vi "load.vi"(8 "error in (no error)":errorcluster, 10 "Node":refnum<k20>, 11 "HP83623A_RF_Generator in":refnum<class "HP83623A_RF_Generator.lvclass">) -> (0 "error out":errorcluster, 2 "node out":refnum<k20>, 3 "HP83623A_RF_Generator out":refnum<class "HP83623A_RF_Generator.lvclass">)   [LabVIEW 2013, in "HP83623A_RF_Generator.lvclass"]
uses:
  HP83623A_RF_Generator.lvclass
  HP83623A.ctl
  HP83623A_RF_Generator.lvclass/HP83623A_RF_Generator.ctl
  <vilib>/xml/Close Reference(Node).vi
  <vilib>/xml/NI_XML.lvlib
  <resource>/objmgr/DOMUserDefRef.rc
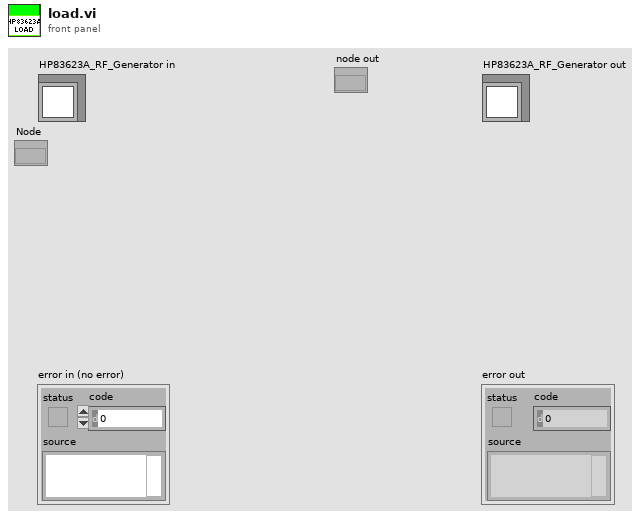
[diagram p1: front panel]
types:
  T1 = typedef "HP83623A_RF_Generator.lvclass/HP83623A.ctl" = cluster{"Frequency (Hz)":dbl, "Power (dBm)":dbl, "Enabled":bool, "initialized":bool, "RF Output On/Off":bool, "External Trigger?":bool, "VISA Session":refnum<visa-resource-name>, "Generator Name":string}
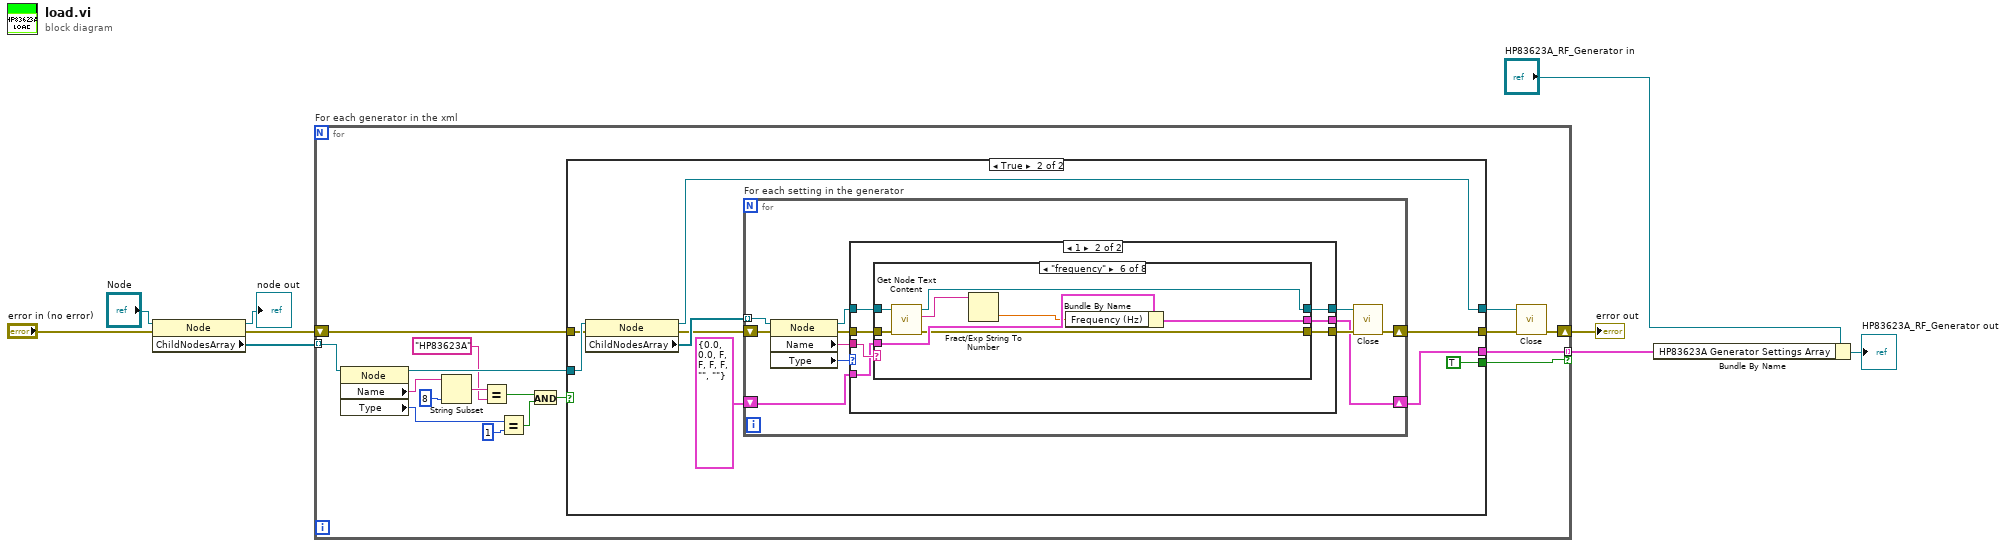
[diagram p0: block diagram]
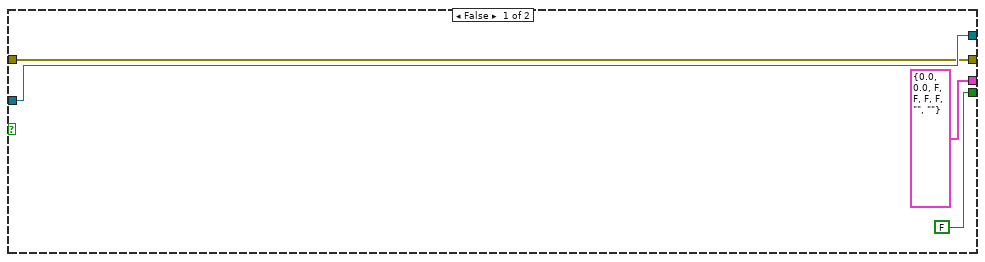
[diagram p2: hidden frame]
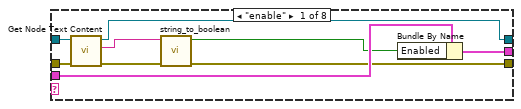
[diagram p4: hidden frame]
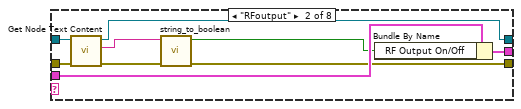
[diagram p5: hidden frame]
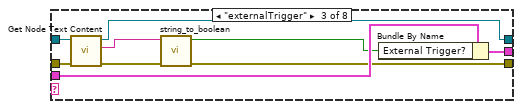
[diagram p6: hidden frame]
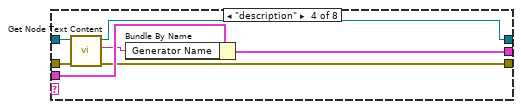
[diagram p7: hidden frame]
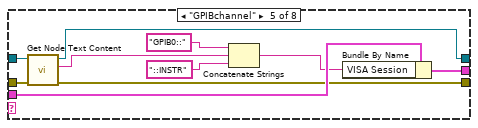
[diagram p8: hidden frame]
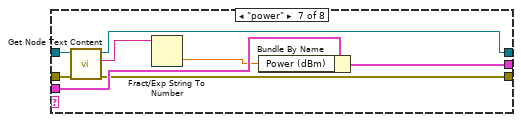
[diagram p9: hidden frame]
diagram:
  n1 = property class="Node"(reference="Node", error in="error in (no error)") -> (reference out=→"node out":refnum<k20>, error out=w1:errorcluster, "ChildNodesArray"=w2:refnum<k20>[])
  n2 = for "For each generator in the xml" {
    tunnel: w2 -> [w21] mode=indexing
    shift-right: [w23] -> w9
    shift-left: w1 -> [w26]
    tunnel: [w10] -> w6 mode=indexing if=w22
    n3 = property class="Node"(reference=w21) -> (reference out=w20:refnum<k20>, "Name"=w16:string, "Type"=w19:i32)  [unwired: 1 in, 1 out]
    n4 = String Subset(string=w16, length (rest)=8 ("length (rest)")) -> (substring=w14:string)  [unwired: 1 in]
    n5 = Equal?(x=w14, y="HP83623A") -> (x = y?=w12:bool)
    n6 = Equal?(x=w19, y=1) -> (x = y?=w17:bool)
    n7 = And(x=w12, y=w17) -> (x .and. y?=w11:bool)
    n8 = case shown="True" w11 {
      tunnel: w20 -> [w30 w39]
      tunnel: w26 -> [w29 w38]
      tunnel: [w30 w35] -> w25
      tunnel: [w29 w34] -> w24
      tunnel: [T1 {"Frequency (Hz)"=0.0, "Power (dBm)"=0.0, "Enabled"=FALSE, "initialized"=FALSE, "RF Output On/Off"=FALSE, "External Trigger?"=FALSE, "VISA Session"="", "Generator Name"=""} ("hp83623a Settings In") w33] -> w10
      tunnel: [FALSE TRUE] -> w22
      frame False {
      }
      frame True {
        n9 = property class="Node"(reference=w39, error in=w38) -> (reference out=w35:refnum<k20>, error out=w36:errorcluster, "ChildNodesArray"=w37:refnum<k20>[])
        n10 = for "For each setting in the generator" {
          shift-right: [w43] -> w34
          shift-left: w36 -> [w47]
          tunnel: w37 -> [w50] mode=indexing
          shift-right: [w41] -> w33
          shift-left: T1 {"Frequency (Hz)"=0.0, "Power (dBm)"=0.0, "Enabled"=FALSE, "initialized"=FALSE, "RF Output On/Off"=FALSE, "External Trigger?"=FALSE, "VISA Session"="", "Generator Name"=""} ("hp83623a Settings In") -> [w42]
          n11 = property class="Node"(reference=w50, error in=w47) -> (reference out=w45:refnum<k20>, error out=w48:errorcluster, "Name"=w49:string, "Type"=w40:i32)
          n12 = case shown="1" w40 {
            tunnel: w49 -> [_ w60]
            tunnel: w48 -> [w52 w59]
            tunnel: [w53 w58] -> w46
            tunnel: w45 -> [w53 w57]
            tunnel: [w52 w56] -> w44
            tunnel: w42 -> [w51 w55]
            tunnel: [w51 w54] -> w41
            frame Default {
            }
            frame 1 {
              n13 = case shown="\"frequency\"" w60 {
                tunnel: w59 -> [w68 w77 w86 w93 w103 w111 w119 w123]
                tunnel: [w61 w70 w79 w88 w99 w107 w115 w123] -> w56
                tunnel: [w65 w74 w83 w89 w100 w108 w116 w122] -> w58
                tunnel: w57 -> [w69 w78 w87 w94 w104 w112 w120 w122]
                tunnel: w55 -> [w67 w76 w85 w92 w102 w110 w118 w121]
                tunnel: [w66 w75 w84 w91 w101 w109 w117 w121] -> w54
                frame "enable" {
                  n14 = call <vilib>:"Get Node Text Content.vi"("error in (no error)"=w68, "node in"=w69) -> ("error out"=w62:errorcluster, "node text"=w64:string, "node out"=w65:refnum<k20>)  [unwired: 7 in]
                  n15 = call "string_to_boolean.vi"("error in"=w62, "string"=w64) -> ("error out"=w61:errorcluster, "boolean"=w63:bool)  [unwired: 8 in]
                  n16 = Bundle By Name(cluster=w67, "Enabled"=w63) -> (w66:T1)
                }
                frame "RFoutput" {
                  n17 = call <vilib>:"Get Node Text Content.vi"("error in (no error)"=w77, "node in"=w78) -> ("error out"=w71:errorcluster, "node text"=w73:string, "node out"=w74:refnum<k20>)  [unwired: 7 in]
                  n18 = call "string_to_boolean.vi"("error in"=w71, "string"=w73) -> ("error out"=w70:errorcluster, "boolean"=w72:bool)  [unwired: 8 in]
                  n19 = Bundle By Name(cluster=w76, "RF Output On/Off"=w72) -> (w75:T1)
                }
                frame "externalTrigger" {
                  n20 = call <vilib>:"Get Node Text Content.vi"("error in (no error)"=w86, "node in"=w87) -> ("error out"=w80:errorcluster, "node text"=w82:string, "node out"=w83:refnum<k20>)  [unwired: 7 in]
                  n21 = call "string_to_boolean.vi"("error in"=w80, "string"=w82) -> ("error out"=w79:errorcluster, "boolean"=w81:bool)  [unwired: 8 in]
                  n22 = Bundle By Name(cluster=w85, "External Trigger?"=w81) -> (w84:T1)
                }
                frame "description" {
                  n23 = call <vilib>:"Get Node Text Content.vi"("error in (no error)"=w93, "node in"=w94) -> ("error out"=w88:errorcluster, "node text"=w90:string, "node out"=w89:refnum<k20>)  [unwired: 7 in]
                  n24 = Bundle By Name(cluster=w92, "Generator Name"=w90) -> (w91:T1)
                }
                frame "GPIBchannel" {
                  n25 = call <vilib>:"Get Node Text Content.vi"("error in (no error)"=w103, "node in"=w104) -> ("error out"=w99:errorcluster, "node text"=w98:string, "node out"=w100:refnum<k20>)  [unwired: 7 in]
                  n26 = Concatenate Strings("GPIB0::" ("string"), w98, "::INSTR" ("string")) -> (w97:string)
                  n27 = Bundle By Name(cluster=w102, "VISA Session"=w97) -> (w101:T1)
                }
                frame "frequency" {
                  n28 = call <vilib>:"Get Node Text Content.vi"("error in (no error)"=w111, "node in"=w112) -> ("error out"=w107:errorcluster, "node text"=w106:string, "node out"=w108:refnum<k20>)  [unwired: 7 in]
                  n29 = Fract/Exp String To Number(string=w106) -> (number=w105:dbl)  [unwired: 3 in, 1 out]
                  n30 = Bundle By Name(cluster=w110, "Frequency (Hz)"=w105) -> (w109:T1)
                }
                frame "power" {
                  n31 = call <vilib>:"Get Node Text Content.vi"("error in (no error)"=w119, "node in"=w120) -> ("error out"=w115:errorcluster, "node text"=w114:string, "node out"=w116:refnum<k20>)  [unwired: 7 in]
                  n32 = Fract/Exp String To Number(string=w114) -> (number=w113:dbl)  [unwired: 3 in, 1 out]
                  n33 = Bundle By Name(cluster=w118, "Power (dBm)"=w113) -> (w117:T1)
                }
                frame Default {
                }
              }
            }
          }
          n34 = call-poly <vilib>:"Close.vi"("error in (no error)"=w44, "node"=w46) -> ("error out"=w43:errorcluster)  [unwired: 7 in]
        }
      }
    }
    n35 = call-poly <vilib>:"Close.vi"("error in (no error)"=w24, "node"=w25) -> ("error out"=w23:errorcluster)  [unwired: 7 in]
  }
  "error out" <- w9
  n36 = Bundle By Name(cluster="HP83623A_RF_Generator in", "HP83623A Generator Settings Array"=w6) -> (→"HP83623A_RF_Generator out":refnum<class "HP83623A_RF_Generator.lvclass">)
